vi "ma_Compute H(w) from IIR Cluster.vi"(0 "IIR Filter Cluster":T1 {"Forward Coefficients" format="%0.4f"; "Reverse Coefficients" format="%0.4f"}, 1 "FFT size":i32=1024) -> (2 "Mag H(w)":dbl[](array[numeric]) format="%0.2f", 3 "Phase H(w)":dbl[](array[numeric]) format="%0.2f", 4 "df":dbl format="%0.2f")   [LabVIEW 2020, in "NI_MAPro.lvlib"]
uses:
  NI_MAPro.lvlib
  NI_AALPro.lvlib
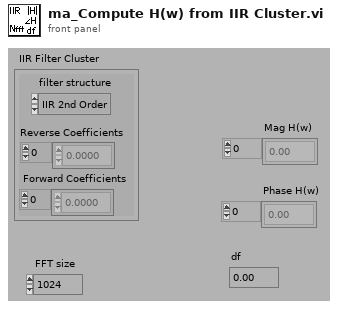
[diagram p1: front panel]
types:
  T1 = cluster{"filter structure":enum32{"IIR 2nd Order", "IIR 4th Order"}, "Reverse Coefficients":dbl[], "Forward Coefficients":dbl[]}
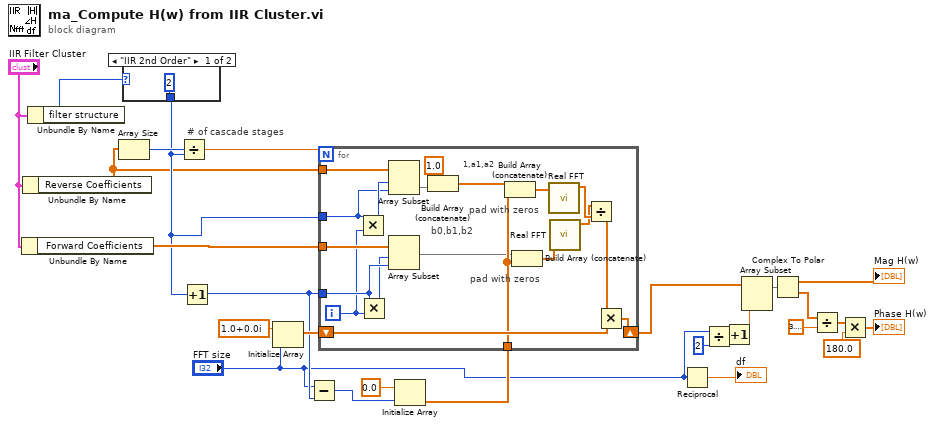
[diagram p0: block diagram]
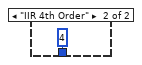
[diagram p2: hidden frame]
diagram:
  # "# of cascade stages"
  n1 = Unbundle By Name("IIR Filter Cluster") -> ("Forward Coefficients"=w24:dbl[])
  n2 = Unbundle By Name("IIR Filter Cluster") -> ("Reverse Coefficients"=w20:dbl[])
  n3 = Unbundle By Name("IIR Filter Cluster") -> ("filter structure"=w26:enum32{"IIR 2nd Order", "IIR 4th Order"})
  n4 = Array Size(array=w20) -> (size(s)=w25:i32)
  n5 = case shown="\"IIR 2nd Order\"" w26 {
    tunnel: [2 4] -> w22
    frame "IIR 2nd Order" {
    }
    frame "IIR 4th Order" {
    }
  }
  n6 = Divide(x=w25, y=w22) -> (x/y=w21:dbl)
  n7 = Increment(x=w22) -> (x+1=w7:i32)
  n8 = Initialize Array(cdb 1.0+0.0i, "FFT size") -> (w18:cdb[])
  n9 = Subtract(x="FFT size", y=w7) -> (x-y=w9:i32)
  n10 = Initialize Array(0.0, w9) -> (w8:dbl[])
  n11 = for {
    N: w21 -> [_]
    shift-right: [w38] -> w13
    shift-left: w18 -> [w36]
    tunnel: w22 -> [w44]
    tunnel: w20 -> [w43]
    tunnel: w24 -> [w42]
    tunnel: w7 -> [w41]
    tunnel: w8 -> [w35]
    i -> [w39]
    # "pad with zeros"
    # "pad with zeros"
    # "b0,b1,b2"
    # "1,a1,a2"
    n12 = Multiply(x=w44, y=w39) -> (x*y=w45:i32)
    n13 = Multiply(x=w41, y=w39) -> (x*y=w40:i32)
    n14 = Array Subset(array=w43, index=w45, length=w44) -> (w47:dbl[])
    n15 = Array Subset(array=w42, index=w40, length=w41) -> (w32:dbl[])
    n16 = Build Array (concatenate)(1.0, w47) -> (w33:dbl[])
    n17 = Build Array (concatenate)(w33, w35) -> (w34:dbl[])
    n18 = Build Array (concatenate)(w32, w35) -> (w31:dbl[])
    n19 = call "Real FFT.vi"("X"=w34) -> ("FFT {X}"=w30:cdb[])  [unwired: 9 in, 1 out]
    n20 = call "Real FFT.vi"("X"=w31) -> ("FFT {X}"=w29:cdb[])  [unwired: 9 in, 1 out]
    n21 = Divide(x=w29, y=w30) -> (x/y=w37:cdb[])
    n22 = Multiply(x=w37, y=w36) -> (x*y=w38:cdb[])
  }
  n23 = Reciprocal(x="FFT size") -> (1/x=→"df":dbl)
  n24 = Divide(x="FFT size", y=2) -> (x/y=w16:dbl)
  n25 = Increment(x=w16) -> (x+1=w15:dbl)
  n26 = Array Subset(array=w13, length=w15) -> (w12:cdb[])  [unwired: 1 in]
  n27 = Complex To Polar(r * e^(i*theta)=w12) -> (r=→"Mag H(w)":dbl[], theta=w2:dbl[])
  n28 = Divide(x=w2, y=3.141592653589793) -> (x/y=w3:dbl[])
  n29 = Multiply(x=w3, y=180.0) -> (x*y=→"Phase H(w)":dbl[])
